vi "MotorControl.vi"(0 "Inputs-statusword":u16, 1 "Inputs-mode_of_operation_display":i8, 2 "halt":bool, 3 "new value":bool, 4 "turn off":bool, 5 "clock":bool) -> (14 "controlword":u16, 15 "Outputs-mode_of_operation":i8, 17 "Status":T1, 18 "Fault":bool, 19 "TargetReached":bool)   [LabVIEW 2020]
uses:
  Statusword_status.ctl
  Modes_out.ctl
  Controlword_transition.ctl
  ElementDTD.lvlib
panel:
  out "Mode_of_operation":T2(ring)
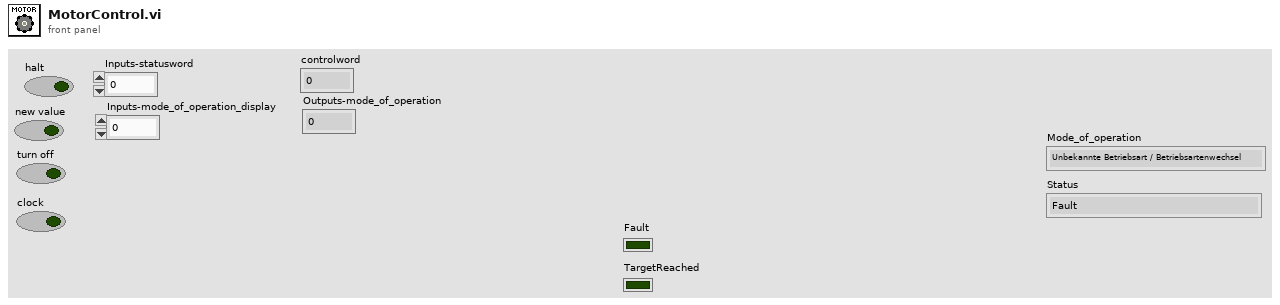
[diagram p1: front panel]
types:
  T1 = typedef "ElementDTD.lvlib/Statusword_status.ctl" = enum16{"Fault", "NOT_READY_TO_SWITCH_ON", "SWITCH_ON_DISABLED", "READY_TO_SWITCH_ON", "SWITCHED_ON", "OPERATION_ENABLE", "QUICK_STOP_ACTIVE"}
  T2 = enum16{"Unbekannte Betriebsart / Betriebsartenwechsel", "User_position_mode", "User_velocity_mode", "User_torque_mode", "Profile_position_mode", "Profile_velocity_mode", "Torque_profile_mode", "Homing_Mode", "Interpolated_position_mode"}
  T3 = typedef "ElementDTD.lvlib/Controlword_transition.ctl" = u16
  T4 = typedef "ElementDTD.lvlib/Modes_out.ctl" = i8
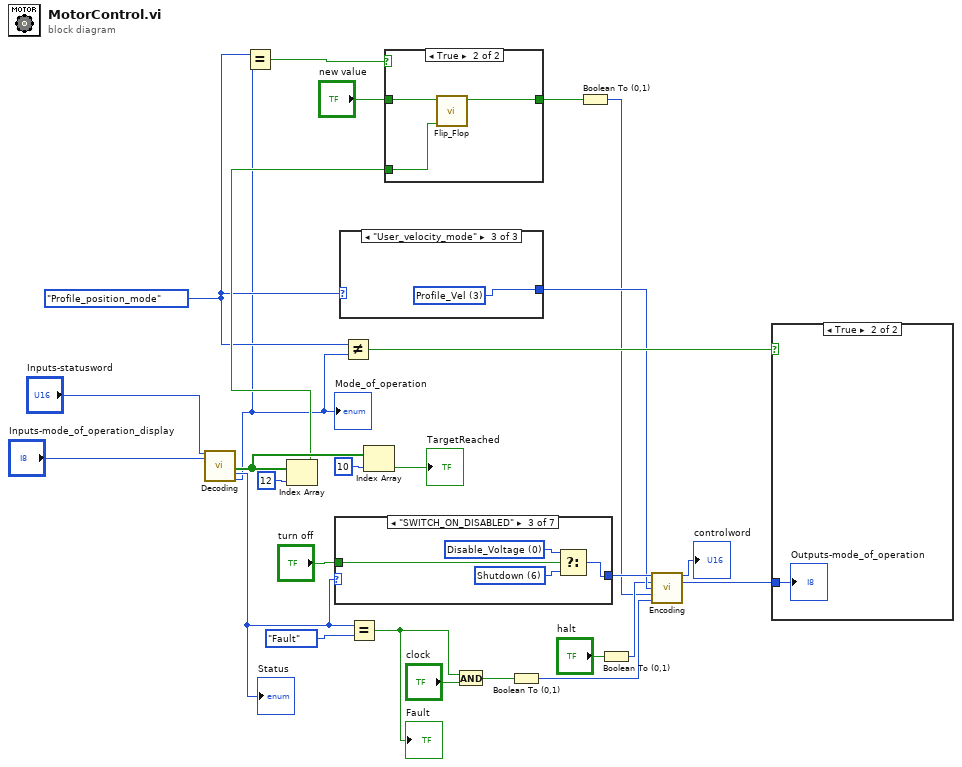
[diagram p0: block diagram]
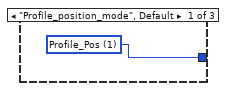
[diagram p3: hidden frame]
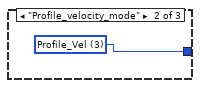
[diagram p4: hidden frame]
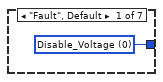
[diagram p6: hidden frame]
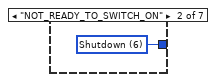
[diagram p7: hidden frame]
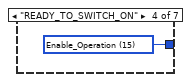
[diagram p8: hidden frame]
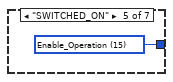
[diagram p9: hidden frame]
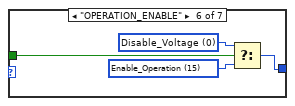
[diagram p10: hidden frame]
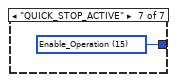
[diagram p11: hidden frame]
diagram:
  w2 = T2."Profile_position_mode" ("Mode_of_operation")
  n1 = call "Decoding.vi"("Inputs-statusword"="Inputs-statusword", "Input-modes_of_operation_display"="Inputs-mode_of_operation_display") -> ("Statusword_out"=w8:bool[], "Status"=w15:T1, "Mode_of_operation"=w1:T2)  [unwired: 15 in]
  "Mode_of_operation" <- w1
  "Status" <- w15
  n2 = Equal?(x=w2, y=w1) -> (x = y?=w7:bool)
  n3 = Index Array(array=w8, index=12 ("Index")) -> (element=w3:bool)
  n4 = case shown="\"SWITCH_ON_DISABLED\"" w15 {
    tunnel: [w28 w29 w32 w34 w35 w37 w40] -> w27
    tunnel: "turn off" -> [_ _ w30 _ _ w36 _]
    frame "Fault", Default {
      w28 = T3 0 items=["Disable_Voltage"=0, "Unknown"=3, "Quick_Stop"=2, "Shutdown"=6, "Enable_Operation"=15] ("transition_out")
    }
    frame "NOT_READY_TO_SWITCH_ON" {
      w29 = T3 6 items=["Disable_Voltage"=0, "Unknown"=3, "Quick_Stop"=2, "Shutdown"=6, "Enable_Operation"=15] ("transition_out")
    }
    frame "SWITCH_ON_DISABLED" {
      w31 = T3 0 items=["Disable_Voltage"=0, "Unknown"=3, "Quick_Stop"=2, "Shutdown"=6, "Enable_Operation"=15] ("transition_out")
      w33 = T3 6 items=["Disable_Voltage"=0, "Unknown"=3, "Quick_Stop"=2, "Shutdown"=6, "Enable_Operation"=15] ("transition_out")
      n5 = Select(t=w31, s=w30, f=w33) -> (s? t:f=w32:T3)
    }
    frame "READY_TO_SWITCH_ON" {
      w34 = T3 15 items=["Disable_Voltage"=0, "Unknown"=3, "Quick_Stop"=2, "Shutdown"=6, "Enable_Operation"=15] ("transition_out")
    }
    frame "SWITCHED_ON" {
      w35 = T3 15 items=["Disable_Voltage"=0, "Unknown"=3, "Quick_Stop"=2, "Shutdown"=6, "Enable_Operation"=15] ("transition_out")
    }
    frame "OPERATION_ENABLE" {
      w39 = T3 0 items=["Disable_Voltage"=0, "Unknown"=3, "Quick_Stop"=2, "Shutdown"=6, "Enable_Operation"=15] ("transition_out")
      w38 = T3 15 items=["Disable_Voltage"=0, "Unknown"=3, "Quick_Stop"=2, "Shutdown"=6, "Enable_Operation"=15] ("transition_out")
      n6 = Select(t=w39, s=w36, f=w38) -> (s? t:f=w37:T3)
    }
    frame "QUICK_STOP_ACTIVE" {
      w40 = T3 15 items=["Disable_Voltage"=0, "Unknown"=3, "Quick_Stop"=2, "Shutdown"=6, "Enable_Operation"=15] ("transition_out")
    }
  }
  n7 = case shown="\"User_velocity_mode\"" w2 {
    tunnel: [w41 w42 w43] -> w24
    frame "Profile_position_mode", Default {
      w41 = T4 1 items=["Profile_Pos"=1, "Profile_Vel"=3, "Torque_Prof"=4, "Homing"=6, "Inter_Pos"=7] ("Mode_out")
    }
    frame "Profile_velocity_mode" {
      w42 = T4 3 items=["Profile_Pos"=1, "Profile_Vel"=3, "Torque_Prof"=4, "Homing"=6, "Inter_Pos"=7] ("Mode_out")
    }
    frame "User_velocity_mode" {
      w43 = T4 3 items=["Profile_Pos"=1, "Profile_Vel"=3, "Torque_Prof"=4, "Homing"=6, "Inter_Pos"=7] ("Mode_out")
    }
  }
  n8 = Not Equal?(x=w2, y=w1) -> (x != y?=w25:bool)
  n9 = Equal?(x=w15, y=Statusword_status."Fault" ("Status")) -> (x = y?=w14:bool)
  "Fault" <- w14
  n10 = Index Array(array=w8, index=10) -> (element=→"TargetReached":bool)
  n11 = case shown="True" w7 {
    tunnel: "new value" -> [w44 w47]
    tunnel: [w44 w45] -> w10
    tunnel: w3 -> [_ w46]
    frame False {
    }
    frame True {
      n12 = call "Flip_Flop.vi"("E1"=w46, "E0"=w47) -> ("A0"=w45:bool)  [unwired: 9 in]
    }
  }
  n13 = And(x=w14, y="clock") -> (x .and. y?=w12:bool)
  n14 = Boolean To (0,1)(Boolean=w12) -> (0, 1=w20:i16)
  n15 = Boolean To (0,1)(Boolean=w10) -> (0, 1=w22:i16)
  n16 = Boolean To (0,1)(Boolean="halt") -> (0, 1=w23:i16)
  n17 = call "Encoding.vi"("transition_out"=w27, "halt"=w23, "Mode_out"=w24, "new_set_point"=w22, "reset"=w20) -> ("controlword"=→"controlword":u16, "Outputs-mode_of_operation"=w26:i8)  [unwired: 9 in]
  n18 = case shown="True" w25 {
    tunnel: w26 -> [_ w48]
    frame False {
    }
    frame True {
      "Outputs-mode_of_operation" <- w48
    }
  }
